vi "Find contact statistic.vi"(0 "reference in":refnum<class "Fcurve.lvclass">, 2 "Deflection (V)":dbl[](array[numeric]), 5 "error in (no error)":errorcluster) -> (14 "reference out":refnum<class "Fcurve.lvclass">, 16 "contact point index out":i32, 19 "error out":errorcluster)   [LabVIEW 2019, in "Fcurve.lvclass"]
doc: "Calculates the index of the contact point by getting the mean and median of the approach portion of the Fcurve, based on std.dev*K (constant)"
uses:
  Fcurve.lvclass
  <vilib>/Analysis/NI_AALBase.lvlib
panel:
  out "mean":dbl format="%0.2f"
  out "variance":dbl format="%0.2f"
  out "Error":bool
  out "size(s)":i32
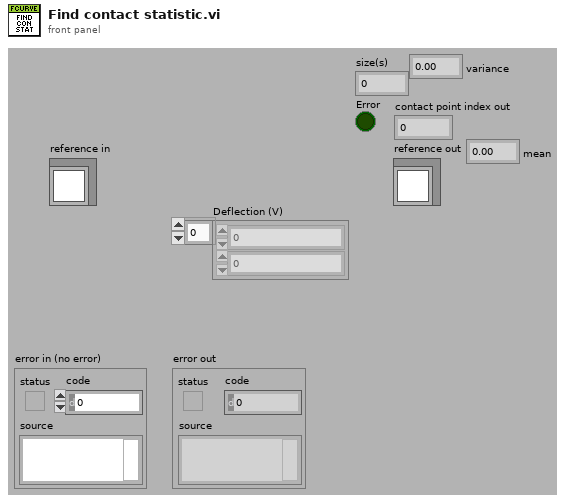
[diagram p1: front panel]
types:
  T1 = typedef "Fcurve.lvclass/ObjectAttributesRef.ctl" = refnum<data-value>
  T2 = typedef "Fcurve.lvclass/ObjectAttributes.ctl" = cluster{"MyAttribute":dbl, "Fcurve Metadata":T3, "Contact Spread of dev":dbl, "Tau Delay (ms)":dbl, "Points of contact":dbl, "Def_wfm":cluster{"Max":dbl, "Min":dbl}, "Zpos_wfm":cluster{"Max":dbl, "Min":dbl}, "Contact stat?":bool, "Real AI dt (s)":dbl, "Decimation":cluster{"App":cluster{"Dec":i32, "apply":bool}, "Con":cluster{"Dec":i32, "apply":bool}, "Ret":cluster{"Dec":i32, "apply":bool}}, "Segment def[0]":dbl, "Segment Zpos[0]":dbl, "Raw Datum":waveform(dbl)[], "Group metadata":T4, "M_data obj":refnum<class "metadata.lvclass">, "Channel name(s)":string[], "Segment fcurve data":cluster{"X":dbl[], "Y":dbl[]}[], "Segment duration":cluster{"Start":i32, "Duration":i32}[], "Segment info":T5[], "Segment durations (S)":dbl[], "Segments Maxmin":T7[]}
  T3 = typedef "Fcurve.lvclass/Metadata.ctl" = cluster{"dt (us)":dbl, "Dec Factor":dbl, "Z piezo Sensitivity (nm/V)":dbl, "K (N/m)":dbl, "Sp (V)":dbl, "Contact (ms)":dbl, "Zpos contact":dbl, "Vel_app (nm/s)":dbl, "Vel_ret (nm/s)":dbl, "deltaV (nm)":dbl, "Def_V0 (v)":dbl, "Piezo gain":dbl, "invOLS (nm/V)":dbl}
  T4 = typedef "TDMS_DataHandler.lvclass/Fcurve Meta data.ctl" = cluster{"property names":string[], "property values":variant[]}
  T5 = typedef "Fcurve.lvclass/Fcurve segments --cluster.ctl" = cluster{"type":T6, "nb points":i32, "dec factor":u32, "sampling rate (S/s)":u32}
  T6 = typedef "metadata.lvclass/Segment type--combobox.ctl" = string
  T7 = typedef "Fcurve.lvclass/Segment MaxMin --cluster.ctl" = cluster{"Def":cluster{"max value":dbl, "min value":dbl}, "Zpos":cluster{"max value":dbl, "min value":dbl}}
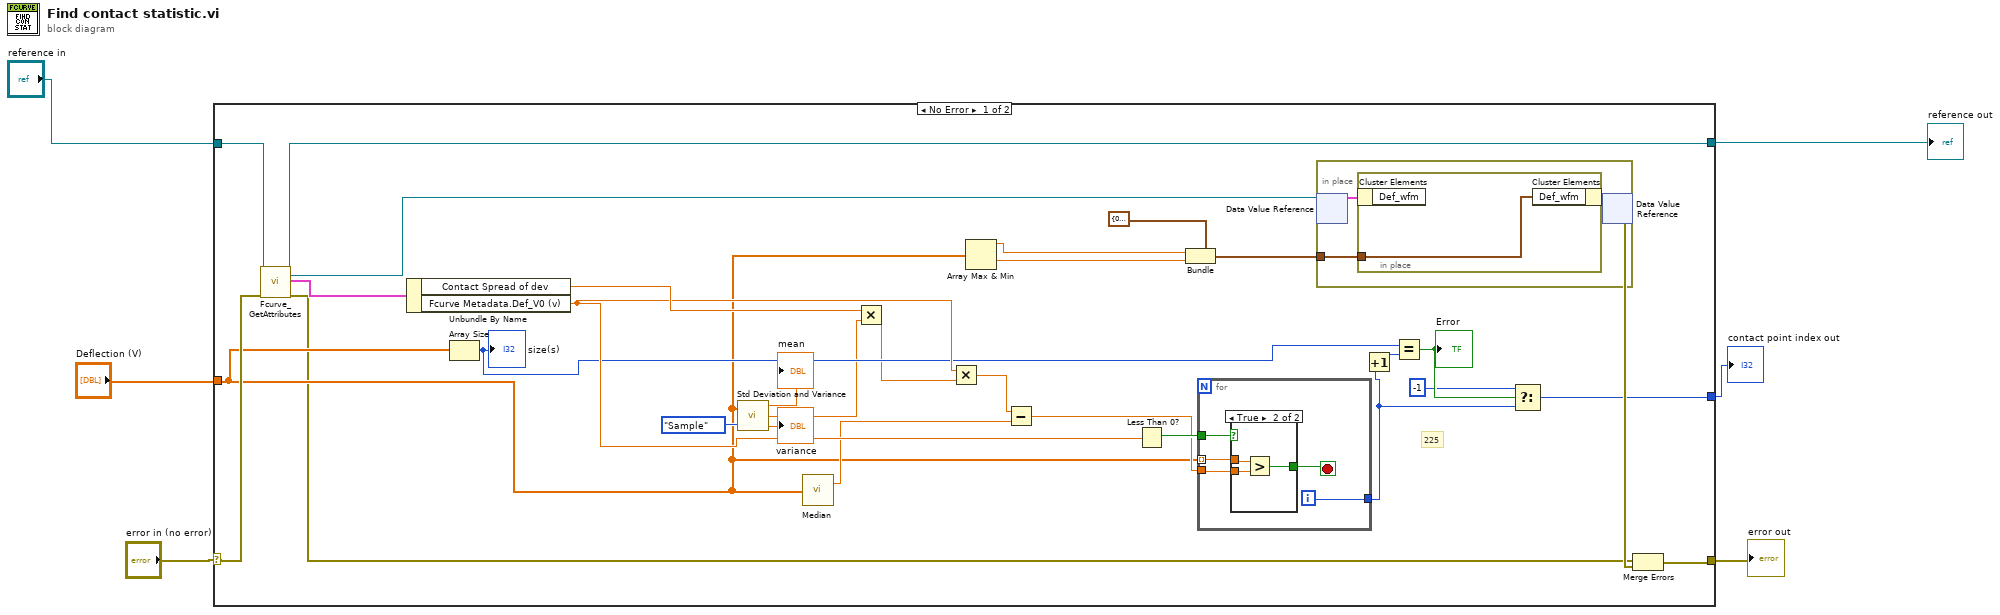
[diagram p0: block diagram]
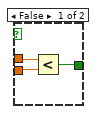
[diagram p2: hidden frame]
diagram:
  n1 = case shown="No Error" "error in (no error)" {
    selector: "error in (no error)" -> [w19 w53]
    tunnel: [w14 w53] -> w6
    tunnel: "reference in" -> [w36 w52]
    tunnel: [w33 w52] -> w4
    tunnel: "Deflection (V)" -> [w18 _]
    tunnel: [w16 _] -> w1
    frame No Error {
      # "225"
      n2 = call "Fcurve_GetAttributes.vi"("reference in"=w36, "error in (no error)"=w19) -> ("reference out"=w33:refnum<class "Fcurve.lvclass">, "attributes ref"=w13:T1, "attributes"=w35:T2, "error out"=w15:errorcluster)  [unwired: 14 in]
      n3 = Unbundle By Name(w35) -> ("Contact Spread of dev"=w34:dbl, "Fcurve Metadata.Def_V0 (v)"=w32:dbl)
      n4 = Array Size(array=w18) -> (size(s)=w31:i32)
      "size(s)" <- w31
      n5 = call <vilib>:"Std Deviation and Variance.vi"("X"=w18, "Weighting (Sample)"=enum16{"Sample", "Population"}."Sample") -> ("mean"=→"mean":dbl, "standard deviation"=w20:dbl, "variance"=→"variance":dbl)
      n6 = call <vilib>:"Median.vi"("X"=w18) -> ("median"=w22:dbl)  [unwired: 1 out]
      n7 = Multiply(x=w34, y=w20) -> (x*y=w21:dbl)
      n8 = Multiply(x=w32, y=w21) -> (x*y=w24:dbl)
      n9 = Array Max & Min(array=w18) -> (max value=w11:dbl, min value=w10:dbl)  [unwired: 2 out]
      n10 = Subtract(x=w24, y=w22) -> (x-y=w23:dbl)
      n11 = Less Than 0?(x=w32) -> (x < 0?=w29:bool)
      n12 = Bundle(cluster=cluster{"Max":dbl, "Min":dbl} {"Max"=0.0, "Min"=0.0} ("Deflection"), "Max"=w11, "Min"=w10) -> (w9:cluster{"Max":dbl, "Min":dbl})
      n13 = for {
        tunnel: w18 -> [w45] mode=indexing
        tunnel: w23 -> [w44]
        tunnel: [w42] -> w28
        tunnel: w29 -> [w41]
        i -> [w42]
        stop <- w43 stop-if-true
        n14 = case shown="True" w41 {
          tunnel: w45 -> [w48 w51]
          tunnel: w44 -> [w47 w50]
          tunnel: [w46 w49] -> w43
          frame False {
            n15 = Less?(x=w48, y=w47) -> (x < y?=w46:bool)
          }
          frame True {
            n16 = Greater?(x=w51, y=w50) -> (0:w49:bool)
          }
        }
      }
      n17 = in-place {
        in-place-border: w9 -> [w37]
        n18 = in-place-dvr #1(w13) -> (w38:T2)  [unwired: 1 out]
        n19 = in-place {
          in-place-border: w37 -> [w40]
          n20 = in-place-cluster #2(w38) -> ()  [unwired: 1 out]
          n21 = in-place-cluster #2("Def_wfm"=w40) -> (w39:T2)
        }
        n22 = in-place-dvr #1(w39) -> (w17:errorcluster)  [unwired: 1 out]
      }
      n23 = Increment(x=w28) -> (x+1=w27:i32)
      n24 = Equal?(x=w31, y=w27) -> (x = y?=w26:bool)
      "Error" <- w26
      n25 = Select(t=-1, s=w26, f=w28) -> (s? t:f=w16:i32)
      n26 = Merge Errors(w15, w17) -> (w14:errorcluster)
    }
    frame Error {
    }
  }
  "error out" <- w6
  "reference out" <- w4
  "contact point index out" <- w1
